vi "SFOAE-Compute OAE Spectra.vi"(0 "DataProc In":T1, 11 "error in (no error)":errorcluster, 13 "Smoothing":cluster{"Length":i32, "Iterations":i32}) -> (4 "DataProc Out":T1, 15 "error out":errorcluster)   [LabVIEW 2020]
uses:
  Typedefs/SFOAE-Data Processing.ctl
  <vilib>/Analysis/baseanly.llb/Mean (DBL).vi
  epl-vi-lib/Utility VIs/Math VIs/dB to Linear (scalar).vi
  epl-vi-lib/Utility VIs/Math VIs/FFT x(t) to dB,Degrees (1D).vi
  epl-vi-lib/Utility VIs/Math VIs/Linear to dB (array).vi
  <vilib>/Analysis/NI_AALBase.lvlib
  <vilib>/Analysis/NI_AALPro.lvlib
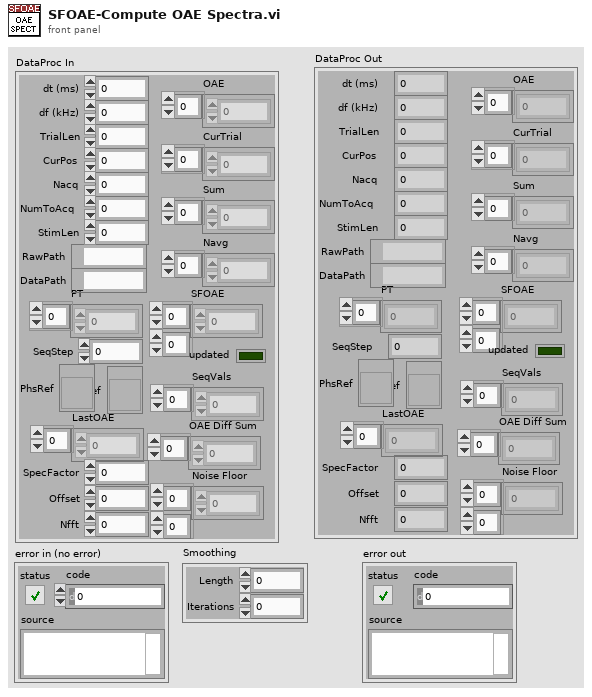
[diagram p1: front panel]
types:
  T1 = typedef "SFOAE-Data Processing.ctl" = cluster{"dt (ms)":dbl, "TrialLen":i32, "PT":cdb[], "CurPos":i32, "Sum":dbl[], "Navg":dbl[], "Nacq":i32, "RawPath":path, "DataPath":path, "NumToAcq":i32, "OAE":dbl[], "CurTrial":dbl[], "StimLen":i32, "SFOAE":cdb[][], "SeqStep":i32, "updated":bool, "SeqVals":dbl[], "df (kHz)":dbl, "MagRef":refnum<vi>, "LastOAE":dbl[], "OAE Diff Sum":dbl[], "Noise Floor":cdb[][], "SpecFactor":dbl, "Offset":i32, "Nfft":i32, "PhsRef":refnum<vi>}
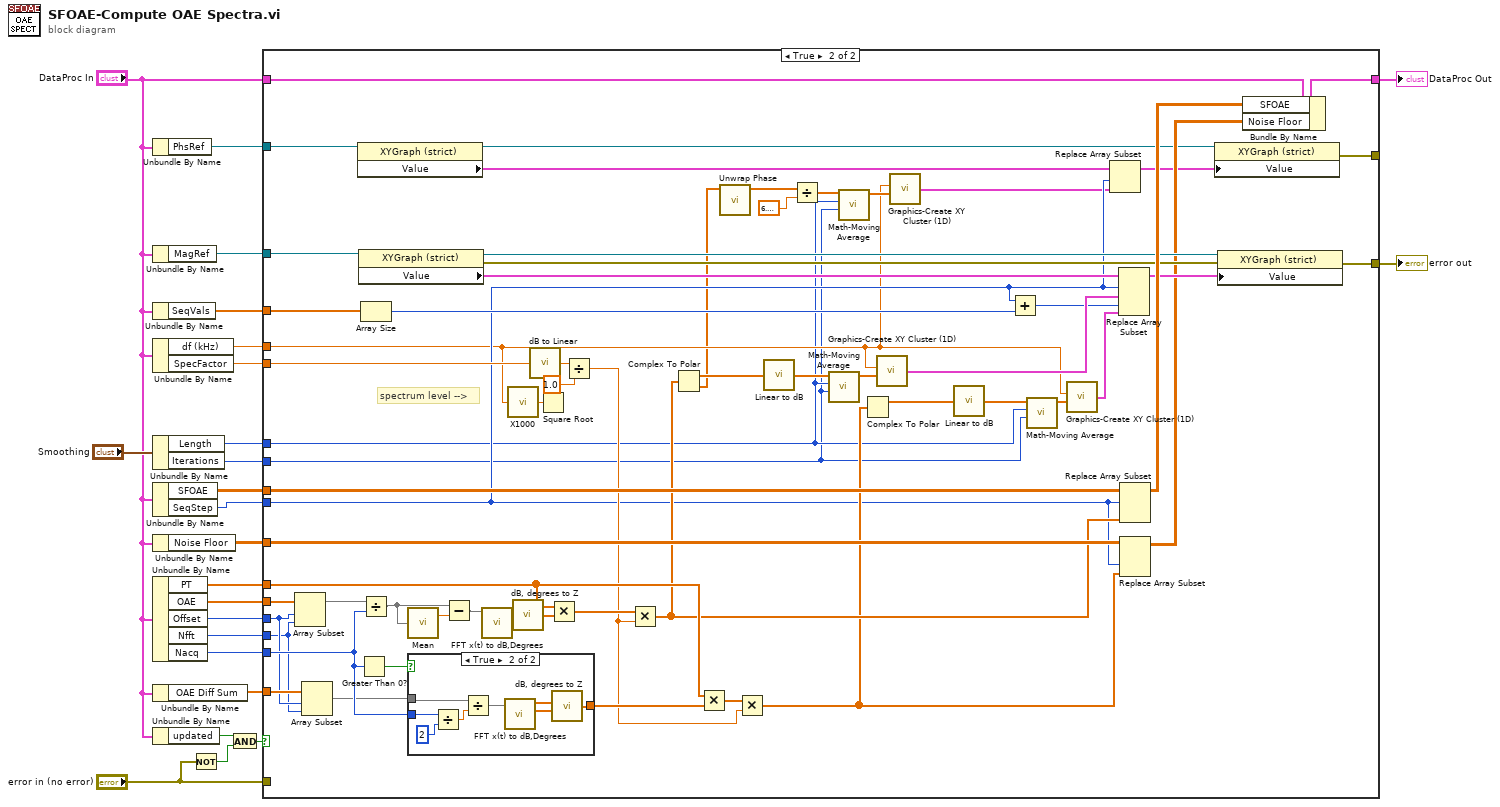
[diagram p0: block diagram]
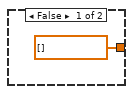
[diagram p3: hidden frame]
diagram:
  n1 = Unbundle By Name("DataProc In") -> ("PhsRef"=w1:refnum<vi>)
  n2 = Unbundle By Name("DataProc In") -> ("MagRef"=w14:refnum<vi>)
  n3 = Unbundle By Name("DataProc In") -> ("SeqVals"=w6:dbl[])
  n4 = Unbundle By Name("DataProc In") -> ("df (kHz)"=w13:dbl, "SpecFactor"=w5:dbl)
  n5 = Unbundle By Name("Smoothing") -> ("Length"=w10:i32, "Iterations"=w9:i32)
  n6 = Unbundle By Name("DataProc In") -> ("SFOAE"=w15:cdb[][], "SeqStep"=w12:i32)
  n7 = Unbundle By Name("DataProc In") -> ("Noise Floor"=w7:cdb[][])
  n8 = Unbundle By Name("DataProc In") -> ("PT"=w16:cdb[], "OAE"=w18:dbl[], "Offset"=w4:i32, "Nfft"=w3:i32, "Nacq"=w17:i32)
  n9 = Unbundle By Name("DataProc In") -> ("OAE Diff Sum"=w8:dbl[])
  n10 = Unbundle By Name("DataProc In") -> ("updated"=w22:bool)
  n11 = Not(x="error in (no error)") -> (.not. x?=w21:bool)
  n12 = And(x=w22, y=w21) -> (x .and. y?=w19:bool)
  n13 = case shown="True" w19 {
    tunnel: "DataProc In" -> [w26 w89]
    tunnel: [w26 w84] -> w23
    tunnel: [w25 w76] -> w24
    tunnel: "error in (no error)" -> [w25 _]
    tunnel: w18 -> [_ w72]
    tunnel: w17 -> [_ w63]
    tunnel: w16 -> [_ w57]
    tunnel: w15 -> [_ w85]
    tunnel: w14 -> [_ w82]
    tunnel: w13 -> [_ w42]
    tunnel: w12 -> [_ w44]
    tunnel: w10 -> [_ w40]
    tunnel: w9 -> [_ w39]
    tunnel: w8 -> [_ w32]
    tunnel: w7 -> [_ w70]
    tunnel: w6 -> [_ w66]
    tunnel: w5 -> [_ w55]
    tunnel: w4 -> [_ w30]
    tunnel: w3 -> [_ w29]
    tunnel: w1 -> [_ w46]
    tunnel: [_ w33] -> _
    frame False {
    }
    frame True {
      # "spectrum level -->"
      n14 = Array Subset(array=w72, index=w30, length=w29) -> (w47:dbl[])
      n15 = Array Subset(array=w32, index=w30, length=w29) -> (w31:dbl[])
      n16 = property class="XYGraph (strict)"(reference=w46) -> (reference out=w35:refnum<vi>, "Value"=w45:cluster{"Array":dbl[], "Array":dbl[]}[])  [unwired: 1 in, 1 out]
      n17 = property class="XYGraph (strict)"(reference=w82) -> (reference out=w77:refnum<vi>, error out=w78:errorcluster, "Value"=w81:cluster{"Array":dbl[], "Array":dbl[]}[])  [unwired: 1 in]
      n18 = Greater Than 0?(x=w63) -> (x > 0?=w73:bool)
      n19 = Array Size(array=w66) -> (size(s)=w64:i32)
      n20 = Divide(x=w47, y=w63) -> (x/y=w59:dbl[])
      n21 = call-poly <vilib>:"Mean.vi"("X"=w59) -> ("mean"=w60:dbl)  [unwired: 1 out]
      n22 = case shown="True" w73 {
        tunnel: w31 -> [_ w98]
        tunnel: [cdb[] [] ("Z") w94] -> w62
        tunnel: w63 -> [_ w93]
        frame False {
        }
        frame True {
          n23 = Divide(x=w93, y=2) -> (x/y=w91:dbl)
          n24 = Divide(x=w98, y=w91) -> (x/y=w95:dbl[])
          n25 = call-poly "FFT x(t) to dB,Degrees.vi"("X"=w95) -> ("+Freq Phase of FFT (degrees)"=w96:dbl[], "+Freq. Mag of FFT (dB rms)"=w97:dbl[])  [unwired: 8 in, 1 out]
          n26 = call "dB, degrees to Z.vi"("Magnitude (dB)"=w97, "Phase (degrees)"=w96) -> ("Z"=w94:cdb[])  [unwired: 5 in]
        }
      }
      n27 = Subtract(x=w59, y=w60) -> (x-y=w58:dbl[])
      n28 = call-poly "FFT x(t) to dB,Degrees.vi"("X"=w58) -> ("+Freq Phase of FFT (degrees)"=w87:dbl[], "+Freq. Mag of FFT (dB rms)"=w88:dbl[])  [unwired: 8 in, 1 out]
      n29 = call "X1000.vi"("X"=w42) -> ("X/1000"=w61:dbl)
      n30 = call "dB, degrees to Z.vi"("Magnitude (dB)"=w88, "Phase (degrees)"=w87) -> ("Z"=w86:cdb[])  [unwired: 5 in]
      n31 = call-poly "dB to Linear.vi"("dB"=w55) -> ("linear"=w54:dbl)
      n32 = Square Root(x=w61) -> ()  [unwired: 1 out]
      n33 = Multiply(x=w57, y=w86) -> (x*y=w80:cdb[])
      n34 = Divide(x=w54, y=1.0) -> (x/y=w52:dbl)
      n35 = Multiply(x=w80, y=w52) -> (x*y=w56:cdb[])
      n36 = Complex To Polar(r * e^(i*theta)=w56) -> (r=w49:dbl[], theta=w37:dbl[])
      n37 = Multiply(x=w57, y=w62) -> (x*y=w68:cdb[])
      n38 = call <vilib>:"Unwrap Phase.vi"("Phase"=w37) -> ("Unwrapped Phase"=w38:dbl[])  [unwired: 9 in, 1 out]
      n39 = Multiply(x=w68, y=w52) -> (x*y=w53:cdb[])
      n40 = call-poly "Linear to dB.vi"("linear"=w49) -> ("dB"=w50:dbl[])
      n41 = Divide(x=w38, y=6.283185307179586) -> (x/y=w36:dbl[])
      n42 = call "Math-Moving Average.vi"("Iterations"=w39, "Length"=w40, "Array in"=w50) -> ("Array out"=w74:dbl[])  [unwired: 8 in]
      n43 = call "Math-Moving Average.vi"("Iterations"=w39, "Length"=w40, "Array in"=w36) -> ("Array out"=w43:dbl[])  [unwired: 8 in]
      n44 = Complex To Polar(r * e^(i*theta)=w53) -> (r=w48:dbl[])  [unwired: 1 out]
      n45 = call "Graphics-Create XY Cluster (1D).vi"("Array"=w74, "dx"=w42) -> ("XY cluster"=w79:cluster{"Array":dbl[], "Array":dbl[]})  [unwired: 2 in]
      n46 = call "Graphics-Create XY Cluster (1D).vi"("Array"=w43, "dx"=w42) -> ("XY cluster"=w41:cluster{"Array":dbl[], "Array":dbl[]})  [unwired: 2 in]
      n47 = call-poly "Linear to dB.vi"("linear"=w48) -> ("dB"=w51:dbl[])
      n48 = Add(x=w44, y=w64) -> (x+y=w65:i32)
      n49 = call "Math-Moving Average.vi"("Iterations"=w39, "Length"=w40, "Array in"=w51) -> ("Array out"=w71:dbl[])  [unwired: 8 in]
      n50 = call "Graphics-Create XY Cluster (1D).vi"("Array"=w71, "dx"=w42) -> ("XY cluster"=w67:cluster{"Array":dbl[], "Array":dbl[]})  [unwired: 2 in]
      n51 = Replace Array Subset(array=w45, new element=w41, index=w44) -> (w34:cluster{"Array":dbl[], "Array":dbl[]}[])
      n52 = Replace Array Subset(array=w81, new element #1=w79, index #1=w44, new element #2=w67, index #2=w65) -> (w75:cluster{"Array":dbl[], "Array":dbl[]}[])
      n53 = Replace Array Subset(array=w85, new element=w56, index (row)=w44) -> (w83:cdb[][])  [unwired: 1 in]
      n54 = Replace Array Subset(array=w70, new element=w53, index (col)=w44) -> (w69:cdb[][])  [unwired: 1 in]
      n55 = property class="XYGraph (strict)"(reference=w35, "Value"=w34) -> (error out=w33:errorcluster)  [unwired: 1 in, 1 out]
      n56 = property class="XYGraph (strict)"(reference=w77, error in=w78, "Value"=w75) -> (error out=w76:errorcluster)  [unwired: 1 out]
      n57 = Bundle By Name(cluster=w89, "SFOAE"=w83, "Noise Floor"=w69) -> (w84:T1)
    }
  }
  "error out" <- w24
  "DataProc Out" <- w23
